vi "Configure Frequency Voltage Range [FVR] Core.vi"(8 "error in (no error)":errorcluster, 10 "freq volt range (10.0 V RMS)":dbl=10.0 format="%^.2e", 11 "IVI_DMM in":refnum<class "IVI_DMM.lvclass">) -> (0 "error out":errorcluster, 3 "IVI_DMM out":refnum<class "IVI_DMM.lvclass">)   [LabVIEW 2015, in "IVI_DMM.lvlib" / "IVI_DMM.lvclass"]
doc: "This VI configures the frequency voltage range of the DMM for frequency and period measurements.\n\nThis VI affects the behavior of the instrument only if the IviDmm>Basic Operation>Function property is set to IVIDMM_VAL_FREQ or IVIDMM_VAL_PERIOD. \n\nNote:\n\n(1) This VI is part of the IviDmmFrequencyMeasurement [FRQ] extension group."
uses:
  IVI_DMM.lvclass
  IVI_DMM.lvclass/IVI_DMM.ctl
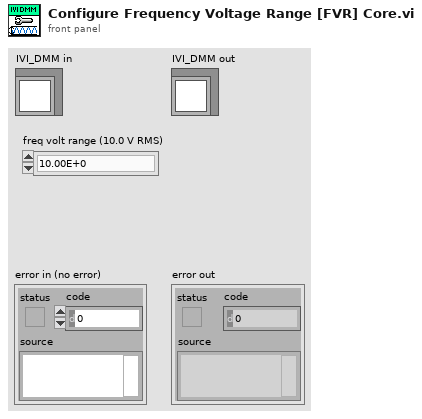
[diagram p1: front panel]
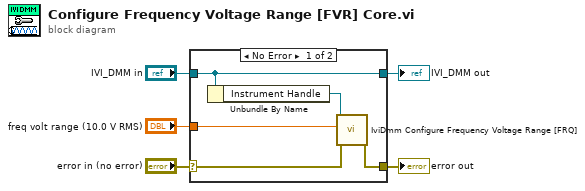
[diagram p0: block diagram]
diagram:
  n1 = case shown="No Error" "error in (no error)" {
    selector: "error in (no error)" -> [w7 w12]
    tunnel: [w9 w12] -> w4
    tunnel: [w10 w11] -> w2
    tunnel: "IVI_DMM in" -> [w10 w11]
    tunnel: "freq volt range (10.0 V RMS)" -> [w6 _]
    frame No Error {
      n2 = Unbundle By Name(w10) -> ("Instrument Handle"=w8:refnum<k15>)
      n3 = call <vilib>:"IviDmm Configure Frequency Voltage Range [FRQ].vi"("error in (no error)"=w7, "freq volt range (10.0 V RMS)"=w6, "instrument handle"=w8) -> ("error out"=w9:errorcluster)  [unwired: 7 in, 1 out]
    }
    frame Error {
    }
  }
  "error out" <- w4
  "IVI_DMM out" <- w2
